vi "SplineHelp_GetQuinticCtrlVectorsFromWayPts.vi"(11 "WayPoints":T1[](array[typedef])) -> (3 "SplineControlVectors":T4[](array[typedef]))   [LabVIEW 2019, in "Trajectory_Library.lvlib"]
doc: "Returns quintic control vectors from a set of waypoints.\n\nParameters:\n - waypoints - The array of waypoints (Translation)\n\nReturns:\n - SplineControlVectors - Array of control vectors"
uses:
  Trajectory_Library.lvlib
  SPLINE_CTRL_VECTOR.ctl
  POSE2D.ctl
  TRANSLATION2D.ctl
  ROTATION2D.ctl
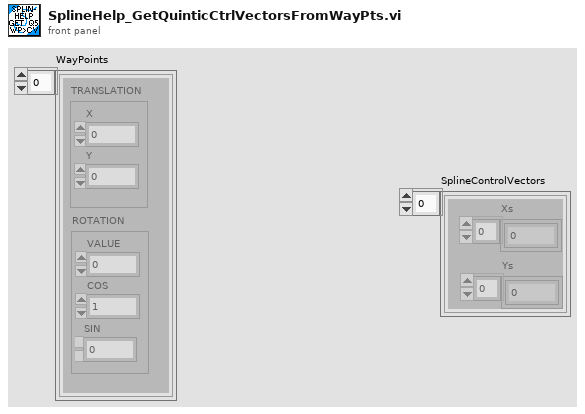
[diagram p1: front panel]
types:
  T1 = typedef "Trajectory_Library.lvlib/POSE2D.ctl" = cluster{"TRANSLATION":T2, "ROTATION":T3}
  T2 = typedef "Trajectory_Library.lvlib/TRANSLATION2D.ctl" = cluster{"X":dbl, "Y":dbl}
  T3 = typedef "Trajectory_Library.lvlib/ROTATION2D.ctl" = cluster{"VALUE":dbl, "COS":dbl, "SIN":dbl}
  T4 = typedef "Trajectory_Library.lvlib/SPLINE_CTRL_VECTOR.ctl" = cluster{"Xs":dbl[], "Ys":dbl[]}
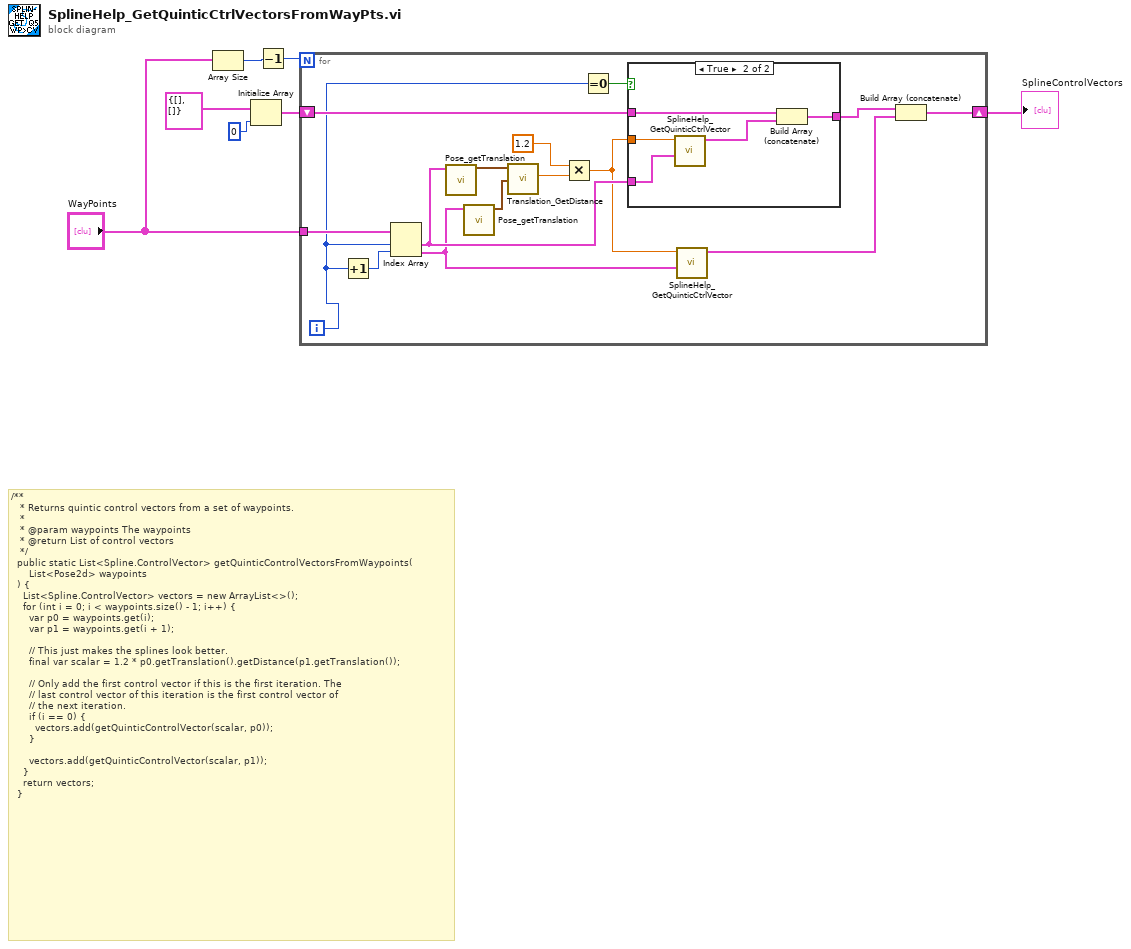
[diagram p0: block diagram]
diagram:
  # "/**\n   * Returns quintic control vectors from a set of waypoints.\n   *\n   * @param waypoints The waypoints\n   * @return List of control vectors\n   */\n  public static List<Spline.ControlVector> getQuinticControlVectorsFromWaypoints(\n      List<Pose2d> waypoints\n  ) {\n    List<Spline.ControlVector> vectors = new ArrayList<>();\n    for (int i = 0; i < waypoints.size() - 1; i++) {\n      var p0 = waypoints.get(i);\n      var p1 = waypoints.get(i + 1);\n\n      // This just makes the splines look better.\n      final var scalar = 1.2 * p0.getTranslation().getDistance(p1.getTranslation());\n\n      // Only add the first control vector if this is the first iteration. The\n      // last control vector of this iteration is the first control vector of\n      // the next iteration.\n      if (i == 0) {\n        vectors.add(getQuinticControlVector(scalar, p0));\n      }\n\n      vectors.add(getQuinticControlVector(scalar, p1));\n    }\n    return vectors;\n  }"
  n1 = Array Size(array="WayPoints") -> (size(s)=w6:i32)
  n2 = Initialize Array(T4 {"Xs"=[], "Ys"=[]} ("SPLINE_CTRL_VECTOR"), 0 ("dimension size")) -> (w3:T4[])
  n3 = Decrement(x=w6) -> (x-1=w7:i32)
  n4 = for {
    N: w7 -> [_]
    tunnel: "WayPoints" -> [w20]
    shift-right: [w12] -> w1
    shift-left: w3 -> [w14]
    i -> [w8]
    n5 = Increment(x=w8) -> (x+1=w21:i32)
    n6 = Index Array(array=w20, index #1=w8, index #2=w21) -> (element #1=w17:T1, element #2=w10:T1)
    n7 = call "Pose_getTranslation.vi"("in POSE"=w17) -> ("outTRANSLATION"=w18:T2)  [unwired: 10 in]
    n8 = call "Pose_getTranslation.vi"("in POSE"=w10) -> ("outTRANSLATION"=w16:T2)  [unwired: 10 in]
    n9 = call "Translation_GetDistance.vi"("other Translation"=w16, "In Translation"=w18) -> ("Distance"=w19:dbl)  [unwired: 9 in]
    n10 = Multiply(x=1.2, y=w19) -> (x*y=w11:dbl)
    n11 = Equal To 0?(x=w8) -> (x = 0?=w15:bool)
    n12 = case shown="True" w15 {
      tunnel: w11 -> [_ w28]
      tunnel: w17 -> [_ w27]
      tunnel: w14 -> [w23 w26]
      tunnel: [w23 w25] -> w13
      frame False {
      }
      frame True {
        n13 = call "SplineHelp_GetQuinticCtrlVector.vi"("Input POSE"=w27, "Scalar"=w28) -> ("resultSpline_Ctrl_Vector"=w24:T4)  [unwired: 9 in]
        n14 = Build Array (concatenate)(w26, w24) -> (w25:T4[])
      }
    }
    n15 = call "SplineHelp_GetQuinticCtrlVector.vi"("Input POSE"=w10, "Scalar"=w11) -> ("resultSpline_Ctrl_Vector"=w9:T4)  [unwired: 9 in]
    n16 = Build Array (concatenate)(w13, w9) -> (w12:T4[])
  }
  "SplineControlVectors" <- w1
